vi "Read Configuration Parameters.vi"(8 "error in (no error)":errorcluster, 10 "refnum":T1, 11 "Example Configuration Dialog in":refnum<class "MotionSystem Configuration.lvclass">) -> (0 "error out":errorcluster, 2 "refnum out":T1, 3 "Example Configuration Dialog out":refnum<class "MotionSystem Configuration.lvclass">)   [LabVIEW 2016, in "MotionSystem.lvlib" / "MotionSystem Configuration.lvclass"]
uses:
  <userlib>/Common Components/Hardware/Abstract System/MotionSystem/MotionSystem Config/MotionSystem Configuration.lvclass
  <vilib>/Utility/config.llb/Config Data RefNum.ctl
  <userlib>/Common Components/Hardware/Abstract System/MotionSystem/MotionSystem Config/SectionName-MotionSystem.ctl
  <userlib>/Common Components/Hardware/Abstract System/MotionSystem/MotionSystem Config/MotionSystem Configuration.lvclass/MotionSystem Configuration.ctl
  <userlib>/Common Components/Hardware/Abstract Hardware/Hardware.lvclass/Hardware.ctl
  <userlib>/Common Components/Hardware/Motor/Motor Config/Motor Configuration.lvclass
  <userlib>/Common Components/Hardware/Abstract Hardware/Read Label.vi
  <userlib>/Common Components/Hardware/Motor/Motor/Motor.lvclass
  C:/Program Files (x86)/National Instruments/LabVIEW 2016/user.lib/Common Components/Hardware/Abstract Hardware/Hardware.lvclass
  <userlib>/Common Components/Hardware/Motor/Motor Config/Accessors/Read Motor Obj.vi
  <userlib>/Common Components/Hardware/Motor/Motor Config/Accessors/Write Motor Obj.vi
  <userlib>/Configuration Dialog Actor/Configuration.lvclass
  <userlib>/Common Components/Hardware/Abstract System/MotionSystem/MotionSystem/MotionSystem.lvclass
  <vilib>/Utility/config.llb/NI_LVConfig.lvlib
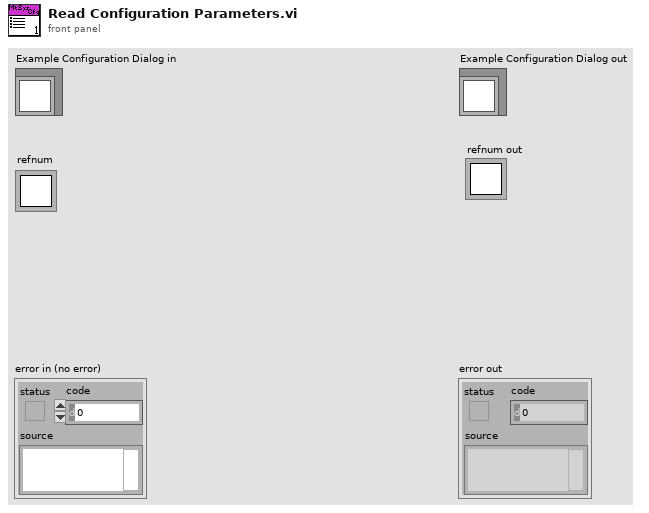
[diagram p1: front panel]
types:
  T1 = typedef "NI_LVConfig.lvlib/Config Data RefNum.ctl" = refnum<k1>
  T2 = typedef "MotionSystem.lvlib/MotionSystem Configuration.lvclass/SectionName-MotionSystem.ctl" = string
  T3 = typedef "MotionSystem.lvlib/MotionSystem Configuration.lvclass/RxRyZ Limits.ctl" = cluster{"Rx (deg)":cluster{"label":string, "soft limit min":dbl, "soft limit max":dbl}, "Ry (deg)":cluster{"label":string, "soft limit min":dbl, "soft limit max":dbl}, "Z (um)":cluster{"label":string, "soft limit min":dbl, "soft limit max":dbl}}
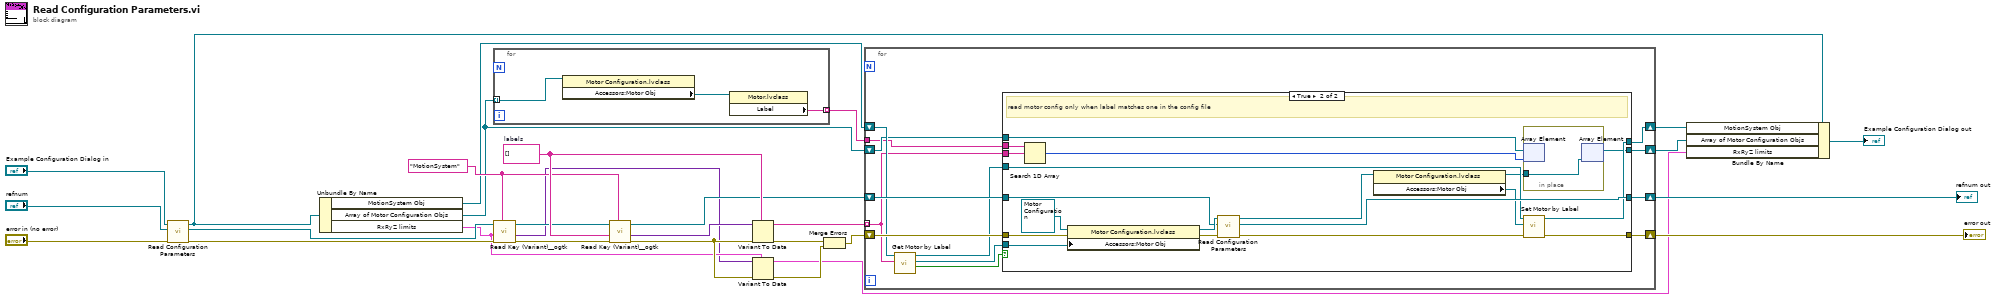
[diagram p0: block diagram]
diagram:
  w26 = string[] []  # labels
  w12 = T2 "MotionSystem"
  n1 = call-parent "Read Configuration Parameters.vi"("error in (no error)"="error in (no error)", "refnum"="refnum", "Configuration in"="Example Configuration Dialog in") -> ("error out"=w19:errorcluster, "refnum out"=w14:T1, "Configuration out"=w16:refnum<class "MotionSystem Configuration.lvclass">)  [unwired: 6 in]
  n2 = Unbundle By Name(w16) -> ("MotionSystem Obj"=w2:refnum<class "MotionSystem.lvclass">, "Array of Motor Configuration Objs"=w1:refnum<class "Motor Configuration.lvclass">[], "RxRyZ limits"=w8:T3)
  n3 = for {
    tunnel: w1 -> [w31] mode=indexing
    tunnel: [w29] -> w20 mode=indexing
    n4 = property class="Motor Configuration.lvclass"(reference=w31) -> ("Accessors:Motor Obj"=w30:refnum<class "Motor.lvclass">)  [unwired: 1 in, 2 out]
    n5 = property class="Motor.lvclass"(reference=w30) -> ("Label"=w29:string)  [unwired: 1 in, 2 out]
  }
  n6 = call <userlib>:"Read Key (Variant)__ogtk.vi"("section"=w12, "error in (no error)"=w19, "type"=w8, "refnum"=w14) -> ("error out"=w15:errorcluster, "key-value"=w7:variant, "refnum out"=w13:T1)  [unwired: 4 in, 1 out]
  n7 = call <userlib>:"Read Key (Variant)__ogtk.vi"("section"=w12, "error in (no error)"=w15, "type"=w26, "refnum"=w13) -> ("error out"=w11:errorcluster, "key-value"=w27:variant, "refnum out"=w24:T1)  [unwired: 4 in, 1 out]
  n8 = Variant To Data(error in=w11, type=w26, Variant=w27) -> (data=w25:string[], error out=w22:errorcluster)
  n9 = Variant To Data(error in=w11, type=w8, Variant=w7) -> (data=w5:T3, error out=w9:errorcluster)
  n10 = Merge Errors(w22, w9) -> (w10:errorcluster)
  n11 = for {
    tunnel: w25 -> [w32] mode=indexing
    shift-right: [w43] -> w23
    shift-left: w24 -> [w44]
    shift-right: [w41] -> w21
    shift-left: w10 -> [w42]
    shift-right: [w36] -> w4
    shift-left: w2 -> [w39]
    shift-right: [w40] -> w3
    shift-left: w1 -> [w34]
    tunnel: w20 -> [w33]
    n12 = call <userlib>:"Get Motor by Label.vi"("label"=w32, "MotionSystem in"=w39) -> ("found"=w35:bool, "Motor obj"=w38:refnum<class "Motor.lvclass">, "MotionSystem out"=w37:refnum<class "MotionSystem.lvclass">)  [unwired: 6 in, 1 out]
    n13 = case shown="True" w35 {
      tunnel: w44 -> [w47 w65]
      tunnel: [w47 w64] -> w43
      tunnel: w42 -> [w46 w62]
      tunnel: [w46 w55] -> w41
      tunnel: [w45 w49] -> w40
      tunnel: w38 -> [_ w60]
      tunnel: w37 -> [w48 w59]
      tunnel: [w48 w57] -> w36
      tunnel: w34 -> [w45 w52]
      tunnel: w33 -> [_ w54]
      tunnel: w32 -> [_ w53]
      frame False {
      }
      frame True {
        # "read motor config only when label matches one in the config file"
        n14 = Search 1D Array(1D array=w54, element=w53) -> (index of element=w51:i32)  [unwired: 1 in]
        n15 = property class="Motor Configuration.lvclass"(reference=refnum<class "Motor Configuration.lvclass"> refnum ("Hardware.lvlib:Motor.lvlib:Motor Configuration.lvclass"), error in=w62, "Accessors:Motor Obj"=w60) -> (reference out=w66:refnum<class "Motor Configuration.lvclass">, error out=w61:errorcluster)
        n16 = call-dynamic "Read Configuration Parameters.vi"("error in (no error)"=w61, "refnum"=w65, "Example Configuration Dialog in"=w66) -> ("error out"=w56:errorcluster, "refnum out"=w64:T1, "Example Configuration Dialog out"=w63:refnum<class "Motor Configuration.lvclass">)  [unwired: 6 in]
        n17 = property class="Motor Configuration.lvclass"(reference=w63) -> (reference out=w50:refnum<class "Motor Configuration.lvclass">, "Accessors:Motor Obj"=w58:refnum<class "Motor.lvclass">)  [unwired: 1 in, 1 out]
        n18 = in-place {
          in-place-border: w50 -> [w68]
          n19 = in-place-array #1(w52, w51) -> ()  [unwired: 1 out]
          n20 = in-place-array #1(w68) -> (w49:refnum<class "Motor Configuration.lvclass">[])  [unwired: 1 out]
        }
        n21 = call <userlib>:"Set Motor by Label.vi"("error in (no error)"=w56, "Motor obj"=w58, "MotionSystem in"=w59) -> ("error out"=w55:errorcluster, "MotionSystem out"=w57:refnum<class "MotionSystem.lvclass">)  [unwired: 7 in]
      }
    }
  }
  "error out" <- w21
  "refnum out" <- w23
  n22 = Bundle By Name(cluster=w16, "MotionSystem Obj"=w4, "Array of Motor Configuration Objs"=w3, "RxRyZ limits"=w5) -> (→"Example Configuration Dialog out":refnum<class "MotionSystem Configuration.lvclass">)
